vi "Calc Load Errors.vi"(10 "[G.Loads]":dbl[](array[numeric]), 11 "[CondyleLoads]":dbl[][](array[numeric])) -> (3 "Load Errors":dbl[][](array[numeric]))   [LabVIEW 2015]
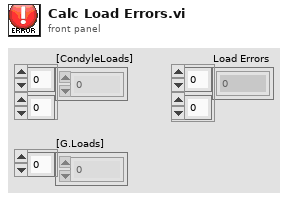
[diagram p1: front panel]
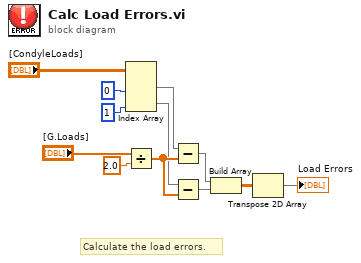
[diagram p0: block diagram]
diagram:
  # "Calculate the load errors."
  n1 = Index Array(array="[CondyleLoads]", index (col) #1=0 ("disabled index (col)"), index (col) #2=1 ("index (col)")) -> (element #1=w4:dbl[], element #2=w5:dbl[])  [unwired: 2 in]
  n2 = Divide(x="[G.Loads]", y=2.0) -> (x/y=w8:dbl[])
  n3 = Subtract(x=w4, y=w8) -> (x-y=w1:dbl[])
  n4 = Subtract(x=w5, y=w8) -> (x-y=w6:dbl[])
  n5 = Build Array(w1, w6) -> (w7:dbl[][])
  n6 = Transpose 2D Array(2D array=w7) -> (transposed array=→"Load Errors":dbl[][])
